vi "sizes_xy.vi"(8 "Size 4":i32, 9 "Size 3":i32, 10 "Size 2":i32, 11 "Size 1":i32) -> (1 "led 1":i32)   [LabVIEW 2011]
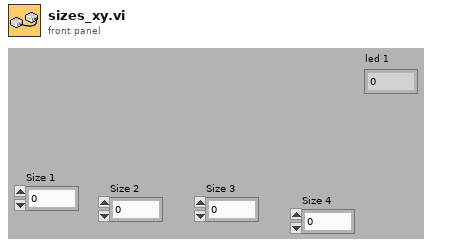
[diagram p1: front panel]
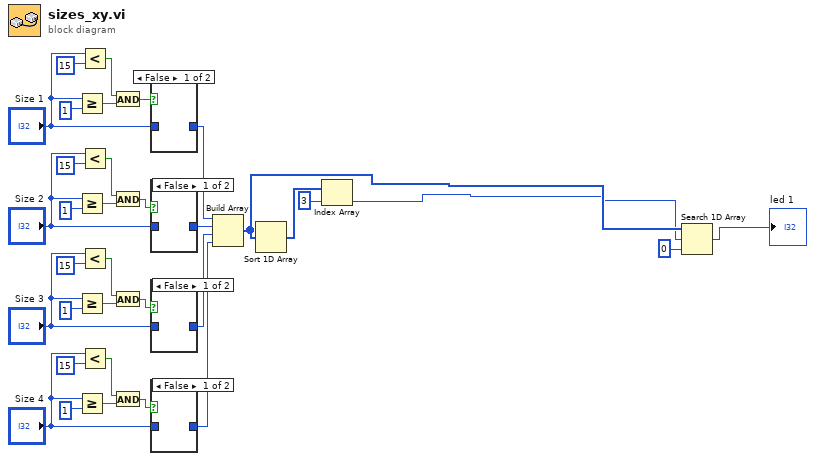
[diagram p0: block diagram]
diagram:
  n1 = Greater Or Equal?(x="Size 1", y=1) -> (x >= y?=w31:bool)
  n2 = Greater Or Equal?(x="Size 2", y=1) -> (x >= y?=w27:bool)
  n3 = Greater Or Equal?(x="Size 3", y=1) -> (x >= y?=w23:bool)
  n4 = Greater Or Equal?(x="Size 4", y=1) -> (x >= y?=w19:bool)
  n5 = Less?(x="Size 1", y=15) -> (x < y?=w32:bool)
  n6 = Less?(x="Size 2", y=15) -> (x < y?=w28:bool)
  n7 = Less?(x="Size 3", y=15) -> (x < y?=w24:bool)
  n8 = Less?(x="Size 4", y=15) -> (x < y?=w20:bool)
  n9 = And(x=w32, y=w31) -> (x .and. y?=w18:bool)
  n10 = And(x=w28, y=w27) -> (x .and. y?=w15:bool)
  n11 = And(x=w24, y=w23) -> (x .and. y?=w8:bool)
  n12 = And(x=w20, y=w19) -> (x .and. y?=w7:bool)
  n13 = case shown="False" w18 {
    tunnel: "Size 1" -> [_ w35]
    tunnel: [_ w35] -> w16
    frame False {
    }
    frame True {
    }
  }
  n14 = case shown="False" w15 {
    tunnel: "Size 2" -> [_ w36]
    tunnel: [_ w36] -> w13
    frame False {
    }
    frame True {
    }
  }
  n15 = case shown="False" w8 {
    tunnel: "Size 3" -> [_ w37]
    tunnel: [_ w37] -> w10
    frame False {
    }
    frame True {
    }
  }
  n16 = case shown="False" w7 {
    tunnel: "Size 4" -> [_ w38]
    tunnel: [_ w38] -> w9
    frame False {
    }
    frame True {
    }
  }
  n17 = Build Array(w16, w13, w10, w9) -> (w4:i32[])
  n18 = Sort 1D Array(array=w4) -> (sorted array=w6:i32[])
  n19 = Index Array(array=w6, index=3) -> (element=w3:i32)
  n20 = Search 1D Array(1D array=w4, element=w3, start index (0)=0) -> (index of element=→"led 1":i32)
